vi "Set Control Attribute To Ini File.vi"(6 "AttributeType":variant, 7 "Section":string, 8 "error in (no error)":errorcluster, 9 "AttributeValue":variant, 10 "AttributeNames":string, 11 "INI Ref":T1) -> (0 "error out":errorcluster, 3 "Ini Ref out":T1)   [LabVIEW 2015, in "UIConfiguration.lvclass"]
uses:
  UIConfiguration.lvclass
  <vilib>/Utility/config.llb/Config Data RefNum.ctl
  <vilib>/Utility/config.llb/Write Key (String).vi
  <vilib>/Utility/config.llb/Write Key (U32).vi
  <vilib>/Utility/config.llb/NI_LVConfig.lvlib
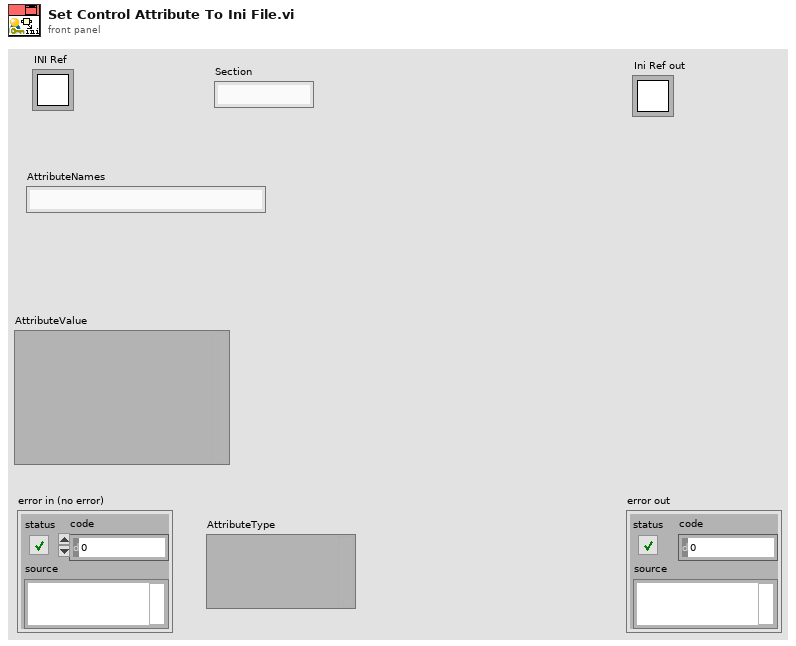
[diagram p1: front panel]
types:
  T1 = typedef "NI_LVConfig.lvlib/Config Data RefNum.ctl" = refnum<k1>
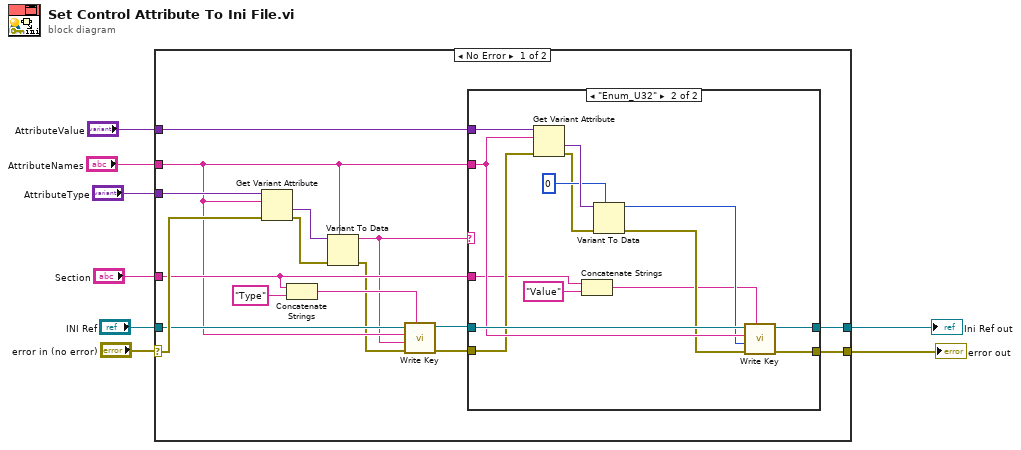
[diagram p0: block diagram]
diagram:
  n1 = case shown="No Error" "error in (no error)" {
    selector: "error in (no error)" -> [w18 w42]
    tunnel: "INI Ref" -> [w15 w41]
    tunnel: "Section" -> [w13 _]
    tunnel: "AttributeType" -> [w23 _]
    tunnel: "AttributeNames" -> [w12 _]
    tunnel: [w20 w41] -> w4
    tunnel: [w19 w42] -> w3
    tunnel: "AttributeValue" -> [w17 _]
    frame No Error {
      n2 = Get Variant Attribute(Variant=w23, name=w12, error in=w18) -> (value=w22:variant, error out=w21:errorcluster)  [unwired: 1 in, 2 out]
      n3 = Concatenate Strings(w13, "Type" ("string")) -> (w14:string)
      n4 = Variant To Data(error in=w21, type=w12, Variant=w22) -> (data=w11:string, error out=w10:errorcluster)
      n5 = call-poly <vilib>:"Write Key.vi"("section"=w14, "error in (no error)"=w10, "value"=w11, "key"=w12, "refnum"=w15) -> ("error out"=w9:errorcluster, "refnum out"=w16:T1)  [unwired: 4 in, 1 out]
      n6 = case shown="\"Enum_U32\"" w11 {
        tunnel: w16 -> [w26 w40]
        tunnel: w9 -> [w25 w37]
        tunnel: w12 -> [_ w38]
        tunnel: w17 -> [_ w39]
        tunnel: [w26 w32] -> w20
        tunnel: [w25 w31] -> w19
        tunnel: w13 -> [_ w28]
        frame Default {
        }
        frame "Enum_U32" {
          n7 = Get Variant Attribute(Variant=w39, name=w38, error in=w37) -> (value=w36:variant, error out=w34:errorcluster)  [unwired: 1 in, 2 out]
          n8 = Concatenate Strings(w28, "Value" ("string")) -> (w27:string)
          n9 = Variant To Data(error in=w34, type=u32 0, Variant=w36) -> (data=w30:u32, error out=w33:errorcluster)
          n10 = call-poly <vilib>:"Write Key.vi"("section"=w27, "error in (no error)"=w33, "value"=w30, "key"=w38, "refnum"=w40) -> ("error out"=w31:errorcluster, "refnum out"=w32:T1)  [unwired: 4 in, 1 out]
        }
      }
    }
    frame Error {
    }
  }
  "Ini Ref out" <- w4
  "error out" <- w3
